vi "Apply force DS345 TDC001 tw.vi"(4 "Moving parameters":T2={"Velocity (mm/s)"=0.5, "Abs position (mm)"=0.0, "Lasting time (s)"=20.0}, 5 "Lasting time (s)":dbl=10.0, 6 "TDC001 motor Serial":i32=83858441, 7 "Apply force":bool, 8 "Cluster":T1={"Osc. Amp. (V)"=0.06, "Osc. Freq. (Hz)"=1200.0} {"Osc. Freq. (Hz)" min=0.001 max=250000.0 step=0.001 format="%.3f"; "Osc. Amp. (V)" min=0.0 max=10.0 step=0.001 format="%.3f"}, 9 "Default setting (DS345)":T1={"Osc. Amp. (V)"=0.01, "Osc. Freq. (Hz)"=1000.0} {"Osc. Freq. (Hz)" min=0.001 max=250000.0 step=0.001 format="%.3f"; "Osc. Amp. (V)" min=0.0 max=0.1 step=0.001 format="%.3f"}, 10 "SRS DS345 GPIB address":string="0:18") -> (0 "Status (s)":dbl)   [LabVIEW 2015]
panel:
  out "Working":bool
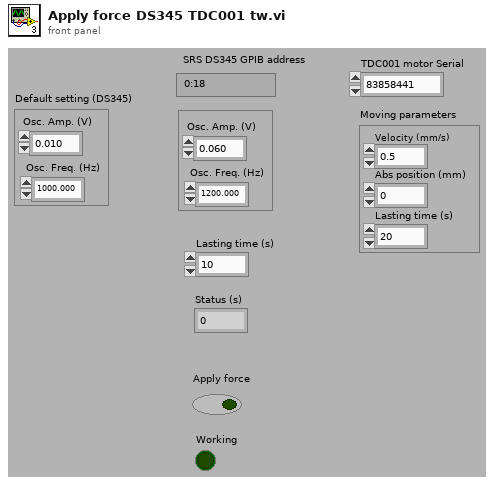
[diagram p1: front panel]
types:
  T1 = cluster{"Osc. Amp. (V)":dbl, "Osc. Freq. (Hz)":dbl}
  T2 = cluster{"Velocity (mm/s)":dbl, "Abs position (mm)":dbl, "Lasting time (s)":dbl}
  T3 = cluster{"Velocity (mm/s)":dbl, dbl, "Lasting time (s)":dbl}
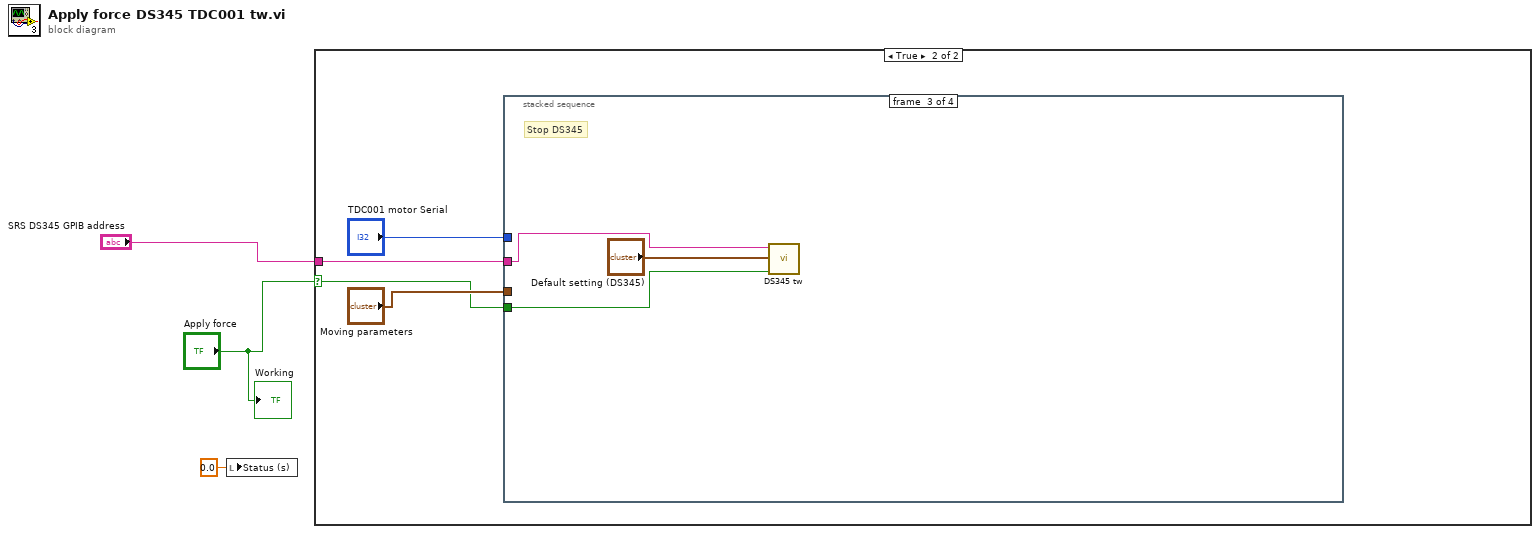
[diagram p0: block diagram]
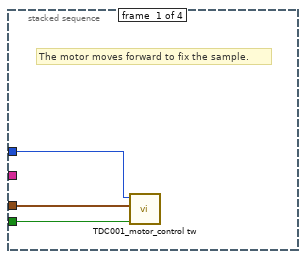
[diagram p3: hidden frame]
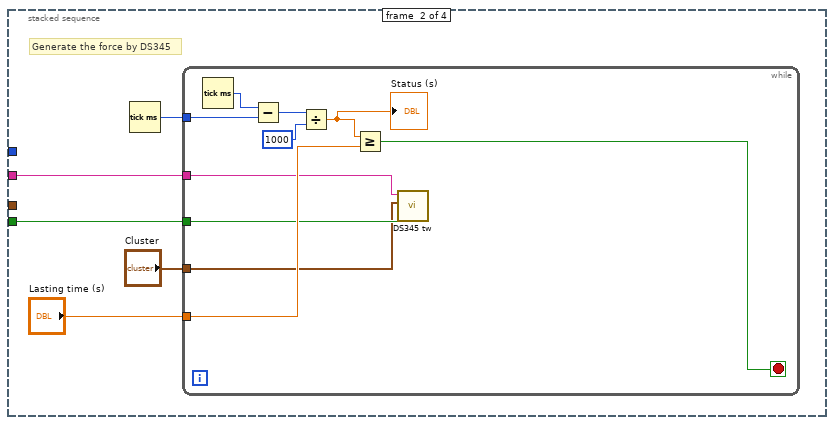
[diagram p4: hidden frame]
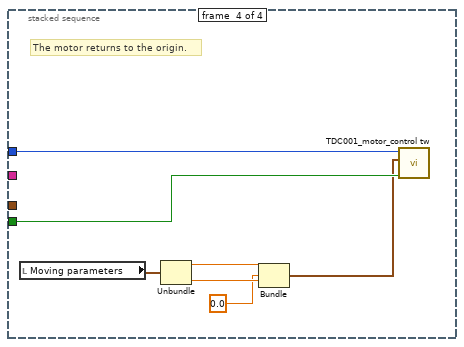
[diagram p5: hidden frame]
diagram:
  n1 = local write "Status (s)"(0.0 ("Status (s)")) -> ()
  n2 = case shown="True" "Apply force" {
    selector: "Apply force" -> [_ w5]
    tunnel: "SRS DS345 GPIB address" -> [_ w4]
    frame False {
    }
    frame True {
      n3 = stacked-sequence {
        tunnel: "TDC001 motor Serial" -> [w10 _ _ w35]
        tunnel: "Moving parameters" -> [w9 _ _ _]
        tunnel: w5 -> [w8 w12 w26 w34]
        tunnel: w4 -> [_ w13 w27 _]
        frame #0 {
          # "The motor moves forward to fix the sample."
          n4 = call "TDC001_motor_control tw.vi"("Move"=w8, "Moving parameters"=w9, "Serial"=w10) -> ()  [unwired: 8 in, 1 out]
        }
        frame #1 {
          # "Generate the force by DS345"
          n5 = Tick Count (ms)() -> (millisecond timer value=w15:u32)
          n6 = while {
            tunnel: w15 -> [w24]
            tunnel: "Lasting time (s)" -> [w20]
            tunnel: w13 -> [w18]
            tunnel: w12 -> [w17]
            tunnel: "Cluster" -> [w16]
            stop <- w23 stop-if-true
            n7 = Tick Count (ms)() -> (millisecond timer value=w25:u32)
            n8 = Subtract(x=w25, y=w24) -> (x-y=w22:u32)
            n9 = Divide(x=w22, y=u32 1000) -> (x/y=w19:dbl)
            "Status (s)" <- w19
            n10 = Greater Or Equal?(x=w19, y=w20) -> (x >= y?=w23:bool)
            n11 = call "DS345 tw.vi"("Update"=w17, "Cluster"=w16, "SRS DS345 GPIB address"=w18) -> ()  [unwired: 9 in]
          }
        }
        frame #2 {
          # "Stop DS345"
          n12 = call "DS345 tw.vi"("Update"=w26, "Cluster"="Default setting (DS345)", "SRS DS345 GPIB address"=w27) -> ()  [unwired: 9 in]
        }
        frame #3 {
          # "The motor returns to the origin."
          n13 = local read "Moving parameters"() -> (w33:T2)
          n14 = Unbundle(w33) -> ("Velocity (mm/s)"=w32:dbl, "Lasting time (s)"=w31:dbl)  [unwired: 1 out]
          n15 = Bundle("Velocity (mm/s)"=w32, 0.0, "Lasting time (s)"=w31) -> (w29:T3)  [unwired: 1 in]
          n16 = call "TDC001_motor_control tw.vi"("Move"=w34, "Moving parameters"=w29, "Serial"=w35) -> ()  [unwired: 8 in, 1 out]
        }
      }
    }
  }
  "Working" <- "Apply force"
